vi "yyllanalysis.vi"(8 "Datain":string[][](array[string]), 11 "StringIN":string) -> (0 "Dataout":string[][](array[string]), 3 "StringOUT":string)   [LabVIEW 2017]
doc: "yyllanalysis是yyll开发的字符串处理指在非编程下处理字符串"
uses:
  yyllanalysis cmd.ctl
  yyllanalysis SettingCtl.ctl
  <vilib>/Utility/miscctls.llb/LVPointTypeDef.ctl
panel:
  in  "Hex?(StringIN)":bool caption="Hex?"
  in  "Hex?(StringOUT)":bool caption="Hex?"
  in  "Hex?(预览)":bool caption="Hex?"
  out "预览":string
  in  "ConfigCluster":T1={"None"={"Nothing to Set"=variant(cluster{"Nothing to Set":variant} {"Nothing to Set"=variant})}, "+CRC"={"CRC"=enum."None", "参与校验起点"=0, "参与校验终点"=999, "CRC16的高低位交换"=FALSE, "发送校验插入点"=999}, "编码运算"={"编码运算"=enum."None", "参与运算数"=0, "移位（正表示顺时搬，右末至左首）"=0}, "提取解析"={"提取"=enum."None", "搜索正则文本"="", "截取起点（负表示向前截取）（不参与正则）"=0, "截取长度（不参与正则）"=999, "源于数据的长度.定位点(U8)"=0, "HEX?(提取搜索文本)"=TRUE}, "数据转换"={"数据转换"=enum."None", "十六进制类型"=enum."U8", "文本类型"=enum."Decimal", "分隔符"="", "分隔符使用"=FALSE}, "增加替换文本"={"增加替换方式"=enum."None", "增加or替换的文本"="", "搜索or正则用的文本"="", "插入点、搜索\\正则匹配点偏移、"=0, "HEX?(增加or替换的文本)"=TRUE, "HEX?(搜索or正则用的文本)"=TRUE}} {"编码运算"."参与运算数" format="%.0b"}
  in  "添加":bool caption="Button"
  in  "删除":bool caption="Button"
  in  "处理方式":T2 caption="Enum 3"
  in  "处理列表":i32(listbox)
  # "yyllanalysis"
  # "#yylltip：如想“D898A2”每2字符间加空格，可用循环正侧匹配增加，搜索正则文本\n设置为“\\w{2}”，增加文本为空格"
  # "#yylltip：分隔符不填会自动使用0x9分割、注意空格是0x20！"
  # "#yylltip：循环正则截取是循环正则处理直到匹配不上，比如“D8:98:A2:8A:B2:0F”\n使用“\\w{2}”输出“D898A28AB20F”;{4}匹配确定的4次;{n,m}最少匹配 n 次且最多匹配 m 次.\n? 等价于 {0,1}。* 等价于 {0,}+ 等价于 {1,}\n源于数据的长度.定位点 是根据原数据某位字节大小来决定截取长度"
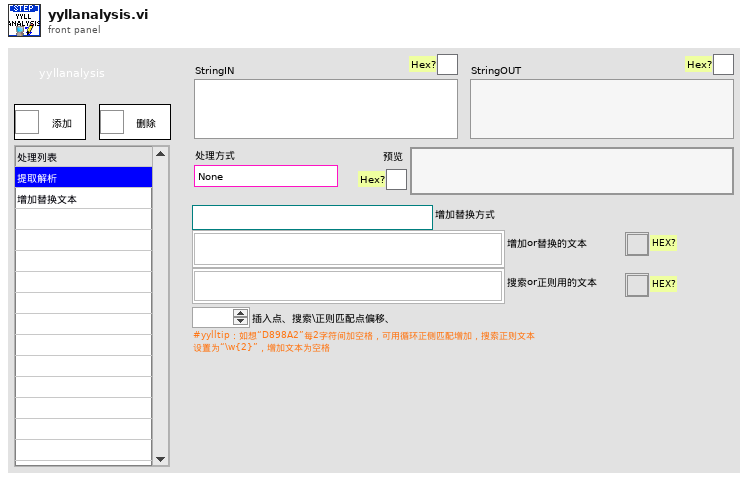
[diagram p1: front panel]
types:
  T1 = typedef "yyllanalysis SettingCtl.ctl" = cluster{"None":cluster{"Nothing to Set":variant}, "+CRC":cluster{"CRC":enum16{"None", "Add8", "CRC-8_CRC-8/SMBUS", "CRC-8_DOW-CRC/MAXIM/MAXIM-DOW", "CRC16_MODBUS", "CRC16_CRC16/ARC/IBM/LHA", "CRC16_XMODEM/ACORN/LTE/V-41-MSB", "CRC16_KERMIT/BLUETOOTH/CCITT/CCITT-TRUE/V-41-LSB", "CRC16_0xFFFF/IBM-3740/AUTOSAR/CCITT-FALSE", "CRC16_GENIBUS/DARC/EPC/EPC-C1G2/I-CODE", "CRC16_0x1D0F/FUJITSU/AUG-CCITT", "CRC32_CRC32/ISO-HDLC/ADCCP/V-42/XZ/PKZIP"}, "参与校验起点":u32, "参与校验终点":u32, "CRC16的高低位交换":bool, "发送校验插入点":u32}, "编码运算":cluster{"编码运算":enum16{"None", "UTF8 to Text", "Text to UTF8", "Reverse翻转", "Trim（）", "与运算", "或运算", "非运算", "右移位（循环）", "计算长度"}, "参与运算数":u64, "移位（正表示顺时搬，右末至左首）":i32}, "提取解析":cluster{"提取":enum16{"None", "固定截取", "固定截取（长度源于数据）", "搜索截取", "正则截取", "循环正则截取"}, "搜索正则文本":string, "截取起点（负表示向前截取）（不参与正则）":i32, "截取长度（不参与正则）":u32, "源于数据的长度.定位点(U8)":i32, "HEX?(提取搜索文本)":bool}, "数据转换":cluster{"数据转换":enum16{"None", "十六进制到文本", "文本到十六进制"}, "十六进制类型":enum16{"U8", "U16", "U32", "U64", "I8", "I16", "I32", "I64", "SGL(4Byte)", "DBL(8Byte)"}, "文本类型":enum16{"Decimal", "Hexadecimal", "Octal"}, "分隔符":string, "分隔符使用":bool}, "增加替换文本":cluster{"增加替换方式":enum16{"None", "固定位增加", "搜索增加", "正则匹配增加", "循环正则匹配增加", "文本替换", "文本替换（全部）"}, "增加or替换的文本":string, "搜索or正则用的文本":string, "插入点、搜索\\正则匹配点偏移、":i32, "HEX?(增加or替换的文本)":bool, "HEX?(搜索or正则用的文本)":bool}}
  T2 = typedef "yyllanalysis cmd.ctl" = enum16{"None", "+CRC", "编码运算", "提取解析", "数据转换", "增加替换文本"}
  T3 = enum16{"open", "replace", "create", "open or create", "replace or create", "replace or create with confirmation"}
  T4 = typedef "LVPointTypeDef.ctl" = cluster{"Horizontal":i16, "Vertical":i16}
  T5 = enum32{"Invalid", "Standard", "Closed", "Hidden", "Minimized", "Maximized"}
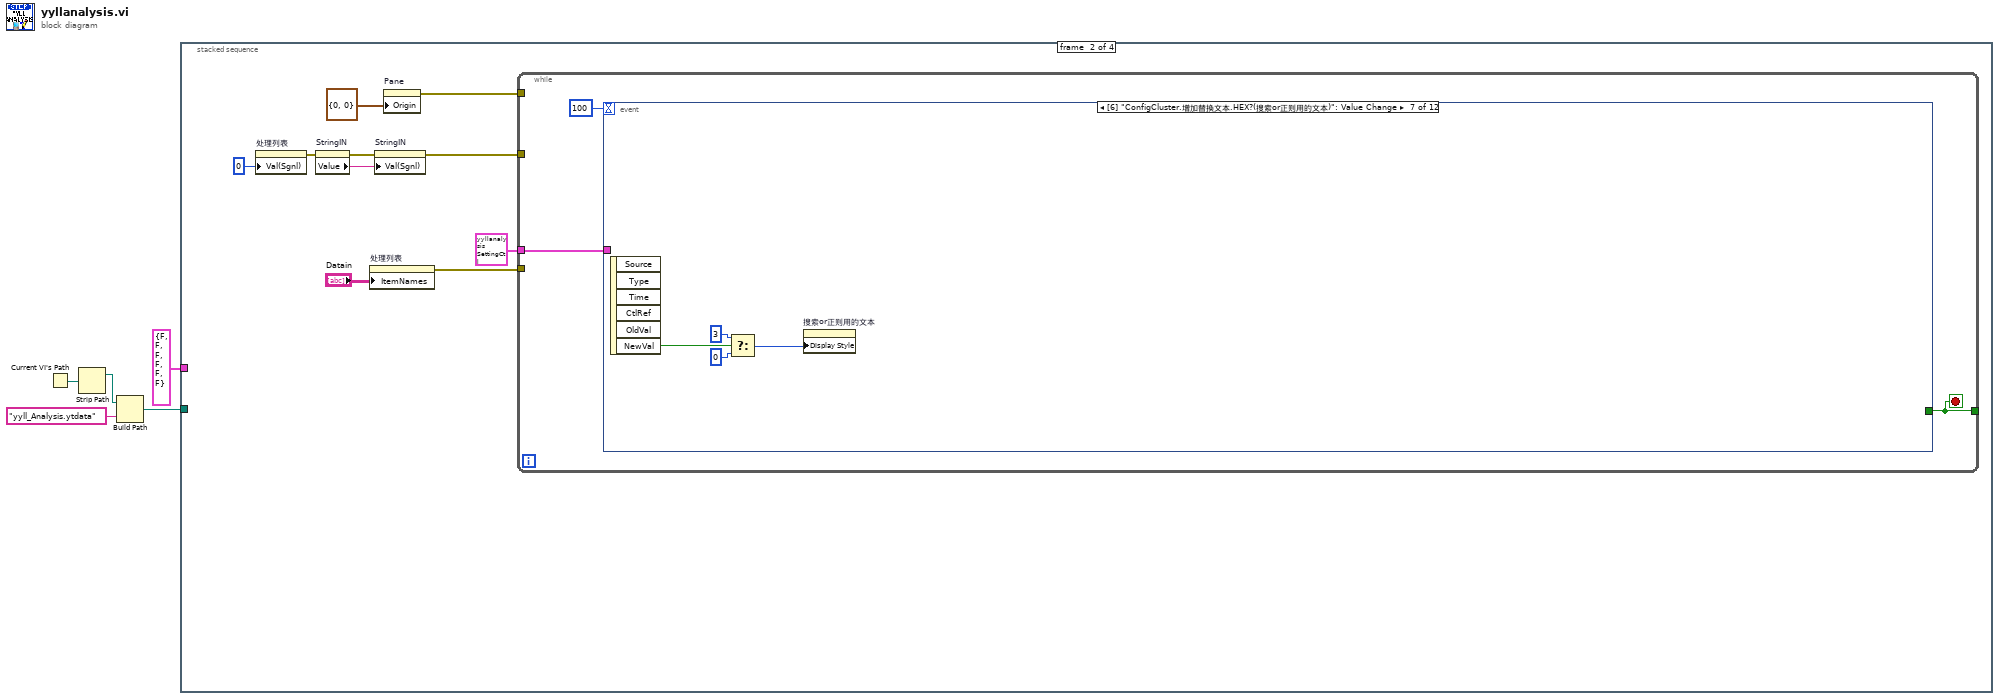
[diagram p0: block diagram]
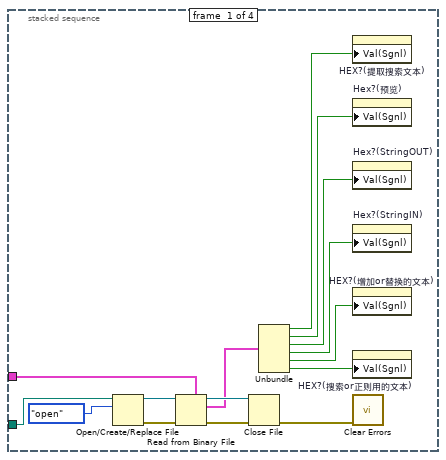
[diagram p2: hidden frame]
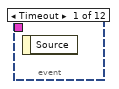
[diagram p3: hidden frame]
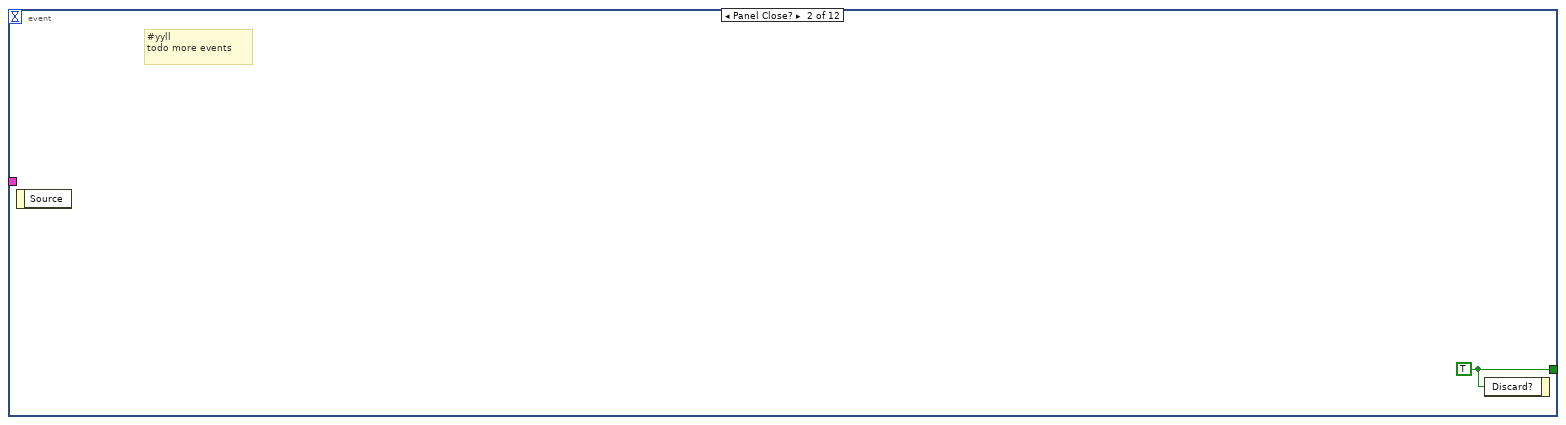
[diagram p4: hidden frame]
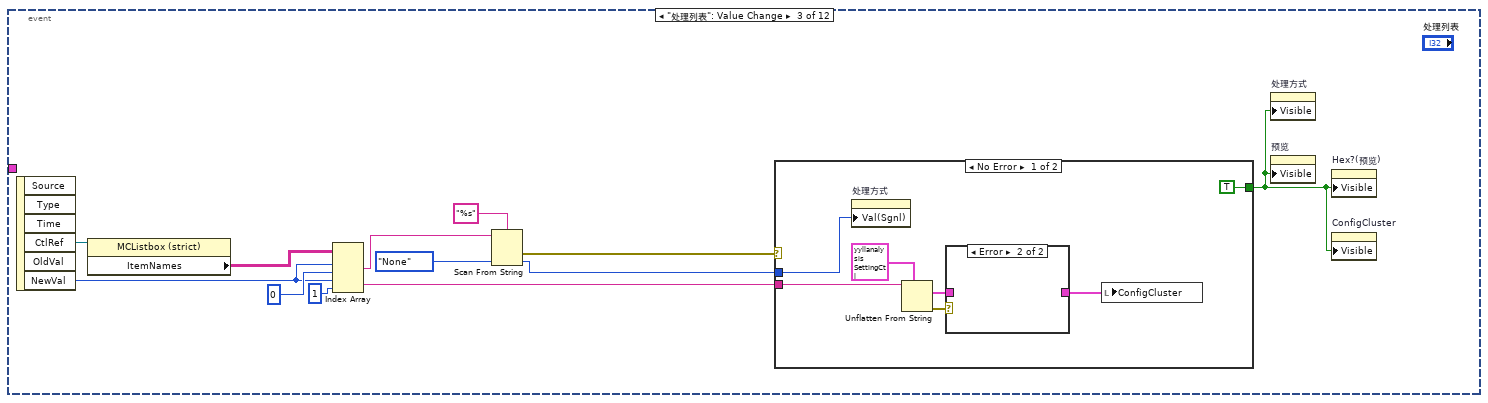
[diagram p5: hidden frame]
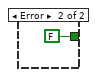
[diagram p7: hidden frame]
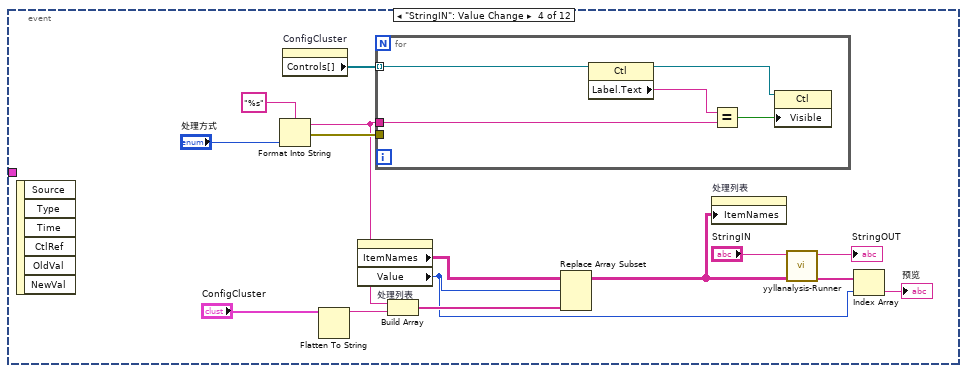
[diagram p8: hidden frame]
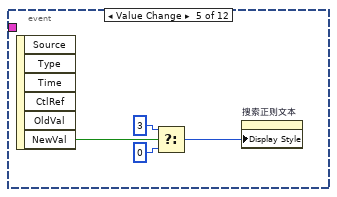
[diagram p9: hidden frame]
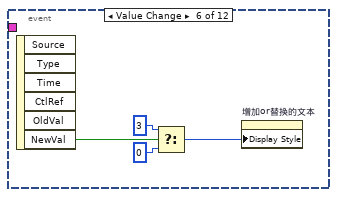
[diagram p10: hidden frame]
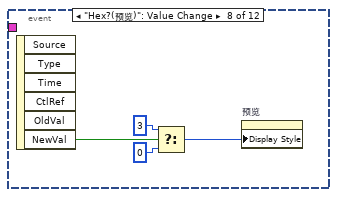
[diagram p11: hidden frame]
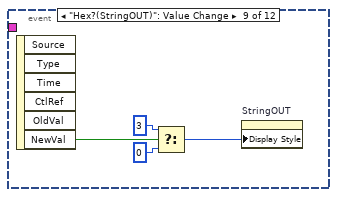
[diagram p12: hidden frame]
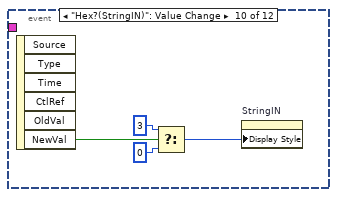
[diagram p13: hidden frame]
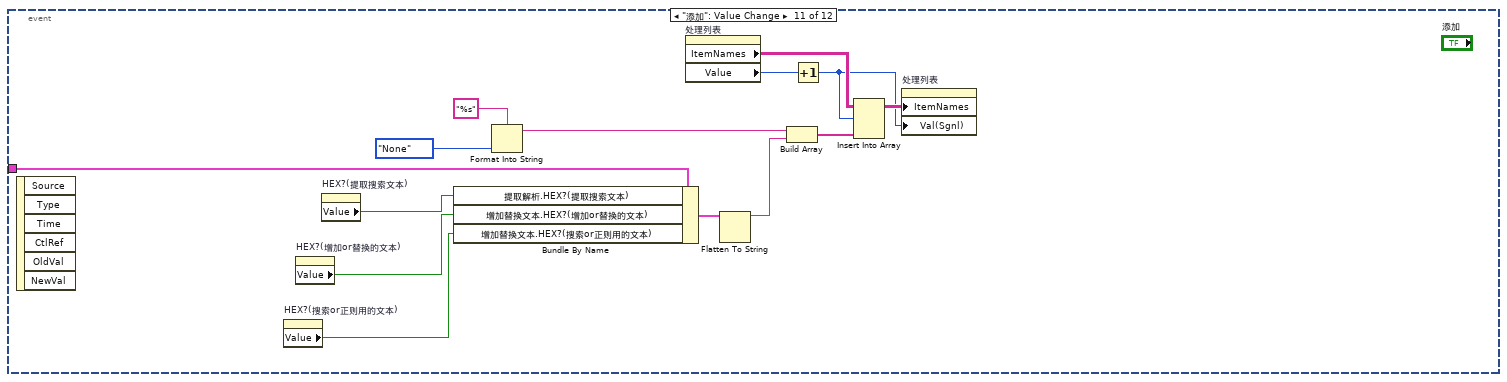
[diagram p14: hidden frame]
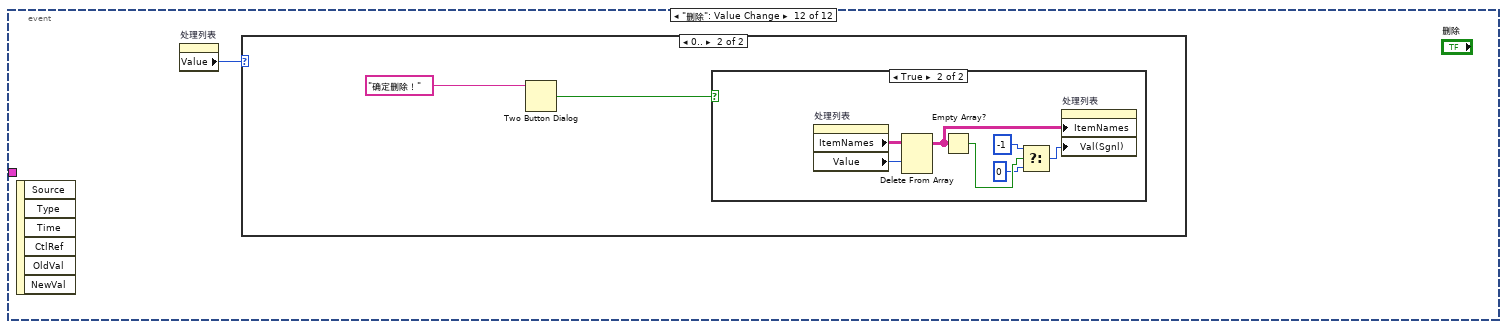
[diagram p15: hidden frame]
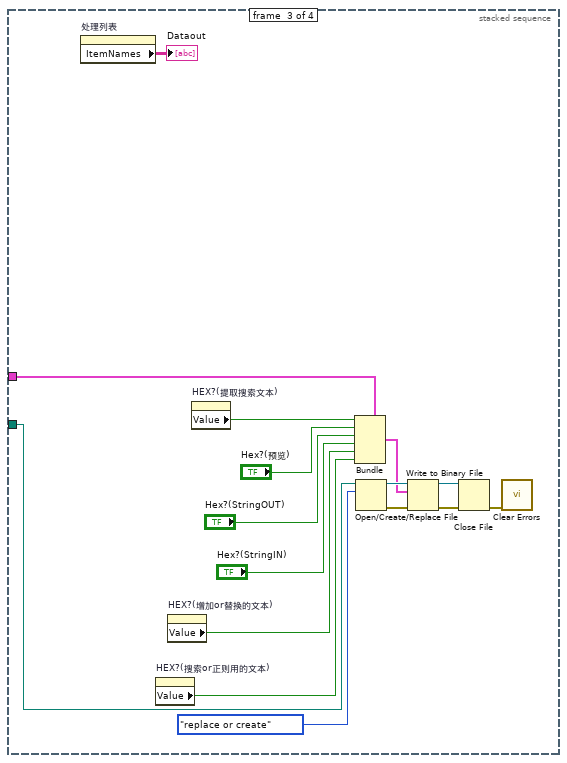
[diagram p18: hidden frame]
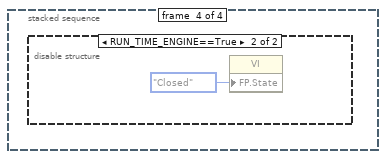
[diagram p19: hidden frame]
diagram:
  n1 = Current VI's Path() -> (path=w3:path)
  n2 = Strip Path(path=w3) -> (stripped path=w4:path)  [unwired: 1 out]
  n3 = Build Path(base path=w4, name or relative path="yyll_Analysis.ytdata") -> (appended path=w2:path)
  n4 = stacked-sequence {
    tunnel: w2 -> [w13 _ w131 _]
    tunnel: cluster{bool, bool, bool, bool, bool, bool} {FALSE, FALSE, FALSE, FALSE, FALSE, FALSE} -> [w12 _ w130 _]
    frame #0 {
      n5 = Open/Create/Replace File(file path (use dialog)=w13, operation (0:open)=T3."open") -> (refnum out=w17:refnum<file>, error out=w15:errorcluster)  [unwired: 4 in, 1 out]
      n6 = Read from Binary File(5:w12, 8:w15, 11:w17) -> (0:w18:errorcluster, 2:w19:cluster{bool, bool, bool, bool, bool, bool}, 3:w20:refnum<file>)  [unwired: 3 in, 1 out]
      n7 = Close File(refnum=w20, error in=w18) -> (error out=w14:errorcluster)  [unwired: 1 out]
      n8 = Unbundle(w19) -> (w11:bool, w10:bool, w9:bool, w8:bool, w7:bool, w6:bool)
      n9 = property on="HEX?(提取搜索文本)" class="Bool (strict)"("Val(Sgnl)"=w11) -> ()  [unwired: 2 in, 2 out]
      n10 = property on="Hex?(预览)" class="Bool (strict)"("Val(Sgnl)"=w10) -> ()  [unwired: 2 in, 2 out]
      n11 = property on="Hex?(StringOUT)" class="Bool (strict)"("Val(Sgnl)"=w9) -> ()  [unwired: 2 in, 2 out]
      n12 = property on="Hex?(StringIN)" class="Bool (strict)"("Val(Sgnl)"=w8) -> ()  [unwired: 2 in, 2 out]
      n13 = property on="HEX?(增加or替换的文本)" class="Bool (strict)"("Val(Sgnl)"=w7) -> ()  [unwired: 2 in, 2 out]
      n14 = property on="HEX?(搜索or正则用的文本)" class="Bool (strict)"("Val(Sgnl)"=w6) -> ()  [unwired: 2 in, 2 out]
      n15 = call <vilib>:"Clear Errors.vi"("error in (no error)"=w14) -> ()  [unwired: 5 in, 2 out]
    }
    frame #1 {
      n16 = property on="处理列表" class="MCListbox (strict)"("Val(Sgnl)"=0 ("Value (Signaling)")) -> (error out=w22:errorcluster)  [unwired: 2 in, 1 out]
      n17 = property on="StringIN" class="Str"(error in=w22) -> (error out=w23:errorcluster, "Value"=w24:string)  [unwired: 1 in, 1 out]
      n18 = property on="处理列表" class="MCListbox (strict)"("ItemNames"="Datain") -> (error out=w27:errorcluster)  [unwired: 2 in, 1 out]
      n19 = property on="StringIN" class="Str"(error in=w23, "Val(Sgnl)"=w24) -> (error out=w21:errorcluster)  [unwired: 1 in, 1 out]
      n20 = property on="Pane" class="Pane"("Origin"=T4 {"Horizontal"=0, "Vertical"=0}) -> (error out=w26:errorcluster)  [unwired: 2 in, 1 out]
      n21 = while {
        tunnel: [w32] -> _
        tunnel: w27 -> [_]
        tunnel: w26 -> [_]
        tunnel: T1 {"None"={"Nothing to Set"=variant(cluster{"Nothing to Set":variant} {"Nothing to Set"=variant})}, "+CRC"={"CRC"=enum."None", "参与校验起点"=0, "参与校验终点"=999, "CRC16的高低位交换"=FALSE, "发送校验插入点"=999}, "编码运算"={"编码运算"=enum."None", "参与运算数"=0, "移位（正表示顺时搬，右末至左首）"=0}, "提取解析"={"提取"=enum."None", "搜索正则文本"="", "截取起点（负表示向前截取）（不参与正则）"=0, "截取长度（不参与正则）"=999, "源于数据的长度.定位点(U8)"=0, "HEX?(提取搜索文本)"=TRUE}, "数据转换"={"数据转换"=enum."None", "十六进制类型"=enum."U8", "文本类型"=enum."Decimal", "分隔符"="", "分隔符使用"=TRUE}, "增加替换文本"={"增加替换方式"=enum."None", "增加or替换的文本"="", "搜索or正则用的文本"="", "插入点、搜索\\正则匹配点偏移、"=0, "HEX?(增加or替换的文本)"=TRUE, "HEX?(搜索or正则用的文本)"=TRUE}} ("ConfigCluster") -> [w31]
        tunnel: w21 -> [_]
        stop <- w32 stop-if-true
        n22 = event shown="[6] \"ConfigCluster.增加替换文本.HEX?(搜索or正则用的文本)\": Value Change" {
          selector: _ -> [_ _ _ _ _ _ _ _ _ _ _ _]
          dyn-events: _ -> [_ _ _ _ _ _ _ _ _ _ _ _]
          timeout: 100 -> [_ _ _ _ _ _ _ _ _ _ _ _]
          tunnel: [_ w34 _ _ _ _ _ _ _ _ _ _] -> w32
          tunnel: w31 -> [_ _ _ _ _ _ _ _ _ _ w104 _]
          event Timeout {
            n23 = event-data() -> ()  [unwired: 1 in, 1 out]
          }
          event Panel Close? {
            w34 = TRUE ("Discard?")
            # "#yyll\ntodo more events"
            n24 = event-data() -> ()  [unwired: 1 in, 1 out]
            n25 = event-data("Discard?"=w34) -> ()  [unwired: 1 in, 1 out]
          }
          event "处理列表": Value Change {
            n26 = event-data() -> ("CtlRef"=w46:refnum<vi>, "NewVal"=w43:i32)  [unwired: 1 in, 4 out]
            n27 = property class="MCListbox (strict)"(reference=w46) -> ("ItemNames"=w45:string[][])  [unwired: 1 in, 2 out]
            n28 = Index Array(array=w45, index (row) #1=w43, index (col) #1=0 ("disabled index (col)"), index (row) #2=w43, index (col) #2=1 ("disabled index (col)")) -> (element #1=w41:string, element #2=w40:string)
            n29 = Scan From String(format string="%s", input string=w41, default 1=yyllanalysis_cmd."None" ("yyllanalysis CMD 2")) -> (error out=w36:errorcluster, output 1=w38:T2)  [unwired: 2 in, 2 out]
            n30 = case shown="No Error" w36 {
              tunnel: w38 -> [w53 _]
              tunnel: w40 -> [w51 _]
              tunnel: [TRUE FALSE] -> w35
              frame No Error {
                n31 = property on="处理方式" class="Enum (strict)"("Val(Sgnl)"=w53) -> ()  [unwired: 2 in, 2 out]
                n32 = Unflatten From String(type=T1 {"None"={"Nothing to Set"=variant(cluster{"Nothing to Set":variant} {"Nothing to Set"=variant})}, "+CRC"={"CRC"=enum."None", "参与校验起点"=0, "参与校验终点"=999, "CRC16的高低位交换"=FALSE, "发送校验插入点"=999}, "编码运算"={"编码运算"=enum."None", "参与运算数"=0, "移位（正表示顺时搬，右末至左首）"=0}, "提取解析"={"提取"=enum."None", "搜索正则文本"="", "截取起点（负表示向前截取）（不参与正则）"=0, "截取长度（不参与正则）"=999, "源于数据的长度.定位点(U8)"=0, "HEX?(提取搜索文本)"=TRUE}, "数据转换"={"数据转换"=enum."None", "十六进制类型"=enum."U8", "文本类型"=enum."Decimal", "分隔符"="", "分隔符使用"=FALSE}, "增加替换文本"={"增加替换方式"=enum."None", "增加or替换的文本"="", "搜索or正则用的文本"="", "插入点、搜索\\正则匹配点偏移、"=0, "HEX?(增加or替换的文本)"=TRUE, "HEX?(搜索or正则用的文本)"=TRUE}} ("ConfigCluster"), binary string=w51) -> (value=w49:T1, error out=w50:errorcluster)  [unwired: 3 in, 1 out]
                n33 = case shown="Error" w50 {
                  tunnel: w49 -> [w54 _]
                  tunnel: [w54 _] -> w48
                  frame No Error {
                  }
                  frame Error {
                  }
                }
                n34 = local write "ConfigCluster"(w48) -> ()
              }
              frame Error {
              }
            }
            n35 = property on="处理方式" class="Enum (strict)"("Visible"=w35) -> ()  [unwired: 2 in, 2 out]
            n36 = property on="预览" class="Str"("Visible"=w35) -> ()  [unwired: 2 in, 2 out]
            n37 = property on="Hex?(预览)" class="Bool (strict)"("Visible"=w35) -> ()  [unwired: 2 in, 2 out]
            n38 = property on="ConfigCluster" class="Clust (strict)"("Visible"=w35) -> ()  [unwired: 2 in, 2 out]
          }
          event "StringIN": Value Change {
            n39 = event-data() -> ()  [unwired: 1 in, 6 out]
            n40 = Format Into String(format string="%s", "处理方式") -> (resulting string=w65:string, error out=w67:errorcluster)  [unwired: 2 in]
            n41 = property on="ConfigCluster" class="Clust (strict)"() -> ("Controls[]"=w70:refnum<vi>[])  [unwired: 2 in, 2 out]
            n42 = Flatten To String(anything="ConfigCluster") -> (data string=w64:string)  [unwired: 3 in, 2 out]
            n43 = property on="处理列表" class="MCListbox (strict)"() -> ("ItemNames"=w63:string[][], "Value"=w57:i32)  [unwired: 2 in, 2 out]
            n44 = for {
              tunnel: w70 -> [w75] mode=indexing
              tunnel: w65 -> [w72]
              tunnel: w67 -> [_]
              n45 = property class="Ctl"(reference=w75) -> (reference out=w74:refnum<vi>, "Label.Text"=w73:string)  [unwired: 1 in, 1 out]
              n46 = Equal?(x=w73, y=w72) -> (x = y?=w71:bool)
              n47 = property class="Ctl"(reference=w74, "Visible"=w71) -> ()  [unwired: 1 in, 2 out]
            }
            n48 = Build Array(w65, w64) -> (w62:string[])
            n49 = Replace Array Subset(array=w63, new element=w62, index (row)=w57) -> (w59:string[][])  [unwired: 1 in]
            n50 = property on="处理列表" class="MCListbox (strict)"("ItemNames"=w59) -> ()  [unwired: 2 in, 2 out]
            n51 = call "yyllanalysis-Runner.vi"("inputs"=w59, "String in"="StringIN") -> ("preview"=w58:string[], "String out"=→"StringOUT":string)  [unwired: 8 in]
            n52 = Index Array(array=w58, index=w57) -> (element=→"预览":string)
          }
          event Value Change {
            n53 = event-data() -> ("NewVal"=w77:bool)  [unwired: 1 in, 5 out]
            n54 = Select(t=u32 3, s=w77, f=u32 0 ("Display Style")) -> (s? t:f=w76:u32)
            n55 = property on="搜索正则文本" class="Str"("Display Style"=w76) -> ()  [unwired: 2 in, 2 out]
          }
          event Value Change {
            n56 = event-data() -> ("NewVal"=w81:bool)  [unwired: 1 in, 5 out]
            n57 = Select(t=u32 3, s=w81, f=u32 0 ("Display Style")) -> (s? t:f=w80:u32)
            n58 = property on="增加or替换的文本" class="Str"("Display Style"=w80) -> ()  [unwired: 2 in, 2 out]
          }
          event Value Change {
            n59 = event-data() -> ("NewVal"=w85:bool)  [unwired: 1 in, 5 out]
            n60 = Select(t=u32 3, s=w85, f=u32 0 ("Display Style")) -> (s? t:f=w84:u32)
            n61 = property on="搜索or正则用的文本" class="Str"("Display Style"=w84) -> ()  [unwired: 2 in, 2 out]
          }
          event "Hex?(预览)": Value Change {
            n62 = event-data() -> ("NewVal"=w88:bool)  [unwired: 1 in, 5 out]
            n63 = Select(t=u32 3, s=w88, f=u32 0 ("Display Style")) -> (s? t:f=w89:u32)
            n64 = property on="预览" class="Str"("Display Style"=w89) -> ()  [unwired: 2 in, 2 out]
          }
          event "Hex?(StringOUT)": Value Change {
            n65 = event-data() -> ("NewVal"=w92:bool)  [unwired: 1 in, 5 out]
            n66 = Select(t=u32 3, s=w92, f=u32 0 ("Display Style")) -> (s? t:f=w93:u32)
            n67 = property on="StringOUT" class="Str"("Display Style"=w93) -> ()  [unwired: 2 in, 2 out]
          }
          event "Hex?(StringIN)": Value Change {
            n68 = event-data() -> ("NewVal"=w96:bool)  [unwired: 1 in, 5 out]
            n69 = Select(t=u32 3, s=w96, f=u32 0 ("Display Style")) -> (s? t:f=w97:u32)
            n70 = property on="StringIN" class="Str"("Display Style"=w97) -> ()  [unwired: 2 in, 2 out]
          }
          event "添加": Value Change {
            n71 = event-data() -> ()  [unwired: 1 in, 6 out]
            n72 = property on="HEX?(搜索or正则用的文本)" class="Bool (strict)"() -> ("Value"=w101:bool)  [unwired: 2 in, 2 out]
            n73 = property on="HEX?(增加or替换的文本)" class="Bool (strict)"() -> ("Value"=w100:bool)  [unwired: 2 in, 2 out]
            n74 = property on="HEX?(提取搜索文本)" class="Bool (strict)"() -> ("Value"=w102:bool)  [unwired: 2 in, 2 out]
            n75 = Bundle By Name(cluster=w104, "提取解析.HEX?(提取搜索文本)"=w102, "增加替换文本.HEX?(增加or替换的文本)"=w100, "增加替换文本.HEX?(搜索or正则用的文本)"=w101) -> (w103:T1)
            n76 = Format Into String(format string="%s", yyllanalysis_cmd."None" ("yyllanalysis CMD 2")) -> (resulting string=w109:string)  [unwired: 2 in, 1 out]
            n77 = property on="处理列表" class="MCListbox (strict)"() -> ("ItemNames"=w113:string[][], "Value"=w106:i32)  [unwired: 2 in, 2 out]
            n78 = Flatten To String(anything=w103) -> (data string=w108:string)  [unwired: 3 in, 2 out]
            n79 = Build Array(w109, w108) -> (w107:string[])
            n80 = Increment(x=w106) -> (x+1=w105:i32)
            n81 = Insert Into Array(array=w113, index (row)=w105, new element=w107) -> (w112:string[][])  [unwired: 1 in]
            n82 = property on="处理列表" class="MCListbox (strict)"("ItemNames"=w112, "Val(Sgnl)"=w105) -> ()  [unwired: 2 in, 2 out]
          }
          event "删除": Value Change {
            n83 = event-data() -> ()  [unwired: 1 in, 6 out]
            n84 = property on="处理列表" class="MCListbox (strict)"() -> ("Value"=w114:i32)  [unwired: 2 in, 2 out]
            n85 = case shown="0.." w114 {
              frame Default {
              }
              frame 0.. {
                n86 = Two Button Dialog(message="确定删除！") -> (T button?=w115:bool)  [unwired: 2 in]
                n87 = case shown="True" w115 {
                  frame False {
                  }
                  frame True {
                    n88 = property on="处理列表" class="MCListbox (strict)"() -> ("ItemNames"=w123:string[][], "Value"=w122:i32)  [unwired: 2 in, 2 out]
                    n89 = Delete From Array(array=w123, index (row)=w122) -> (array with subset deleted=w121:string[][])  [unwired: 2 in, 1 out]
                    n90 = Empty Array?(array=w121) -> (empty?=w120:bool)
                    n91 = Select(t=-1 ("Value (Signaling)"), s=w120, f=0 ("Value (Signaling)")) -> (s? t:f=w117:i32)
                    n92 = property on="处理列表" class="MCListbox (strict)"("ItemNames"=w121, "Val(Sgnl)"=w117) -> ()  [unwired: 2 in, 2 out]
                  }
                }
              }
            }
          }
        }
      }
    }
    frame #2 {
      n93 = property on="处理列表" class="MCListbox (strict)"() -> ("ItemNames"=→"Dataout":string[][])  [unwired: 2 in, 2 out]
      n94 = property on="HEX?(搜索or正则用的文本)" class="Bool (strict)"() -> ("Value"=w124:bool)  [unwired: 2 in, 2 out]
      n95 = property on="HEX?(增加or替换的文本)" class="Bool (strict)"() -> ("Value"=w125:bool)  [unwired: 2 in, 2 out]
      n96 = property on="HEX?(提取搜索文本)" class="Bool (strict)"() -> ("Value"=w139:bool)  [unwired: 2 in, 2 out]
      n97 = Bundle(cluster=w130, w139, "Hex?(预览)", "Hex?(StringOUT)", "Hex?(StringIN)", w125, w124) -> (w135:cluster{bool, bool, bool, bool, bool, bool})
      n98 = Open/Create/Replace File(file path (use dialog)=w131, operation (0:open)=T3."replace or create") -> (refnum out=w136:refnum<file>, error out=w137:errorcluster)  [unwired: 4 in, 1 out]
      n99 = Write to Binary File(file (use dialog)=w136, data=w135, error in=w137) -> (refnum out=w133:refnum<file>, error out=w134:errorcluster)  [unwired: 3 in, 1 out]
      n100 = Close File(refnum=w133, error in=w134) -> (error out=w138:errorcluster)  [unwired: 1 out]
      n101 = call <vilib>:"Clear Errors.vi"("error in (no error)"=w138) -> ()  [unwired: 5 in, 2 out]
    }
    frame #3 {
      n102 = disable-structure shown="RUN_TIME_ENGINE==True" {
        frame condition #0 (active) {
        }
        frame condition #1 {
          n103 = property class="VI"("FP.State"=T5."Closed" ("前面板窗口:状态")) -> ()  [unwired: 2 in, 2 out]
        }
      }
    }
  }
